vi "stiffnessSummaryView.vi"(10 "UserEvents in":refnum<class "UserEvents.lvclass">) -> ()   [LabVIEW 2015, in "M1M3SSSTViews.lvlib"]
uses:
  M1M3SSSTViews.lvlib
  UserEvents/UserEvents.lvclass
  UserEvents/UserEvents.lvclass/UserEvents.ctl
  Typedefs/StateSelector.ctl
  Typedefs/M1M3SSSTypedefs.lvlib
panel:
  in  "Stiffnesses Summary":string[][](table)
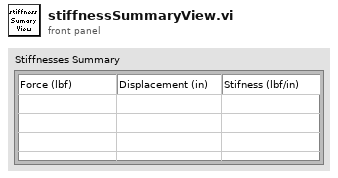
[diagram p1: front panel]
types:
  T1 = typedef "M1M3SSSTypedefs.lvlib/PubDataEvents.ctl" = cluster{"State":refnum<user-event>, "ErrorCode":refnum<user-event>, "OutputData":refnum<user-event>, "InputData":refnum<user-event>, "ControllerData":refnum<user-event>, "TestStatus":refnum<user-event>, "LogPath":refnum<user-event>, "StiffnessDataAssembly":refnum<user-event>, "PreconditioningCycle":refnum<user-event>}
  T2 = cluster{"Event Registration Refnum":refnum<event-registration>, "Event Registration Refnum":refnum<event-registration>}
  T3 = typedef "M1M3SSSTypedefs.lvlib/StateSelector.ctl" = enum16{"FaultState", "OffState", "RampingUpPressurePState", "RampingUpPressureSTState", "StandbyState", "StoppedState", "WaitingForSettledPState", "WaitingForSettledSTState"}
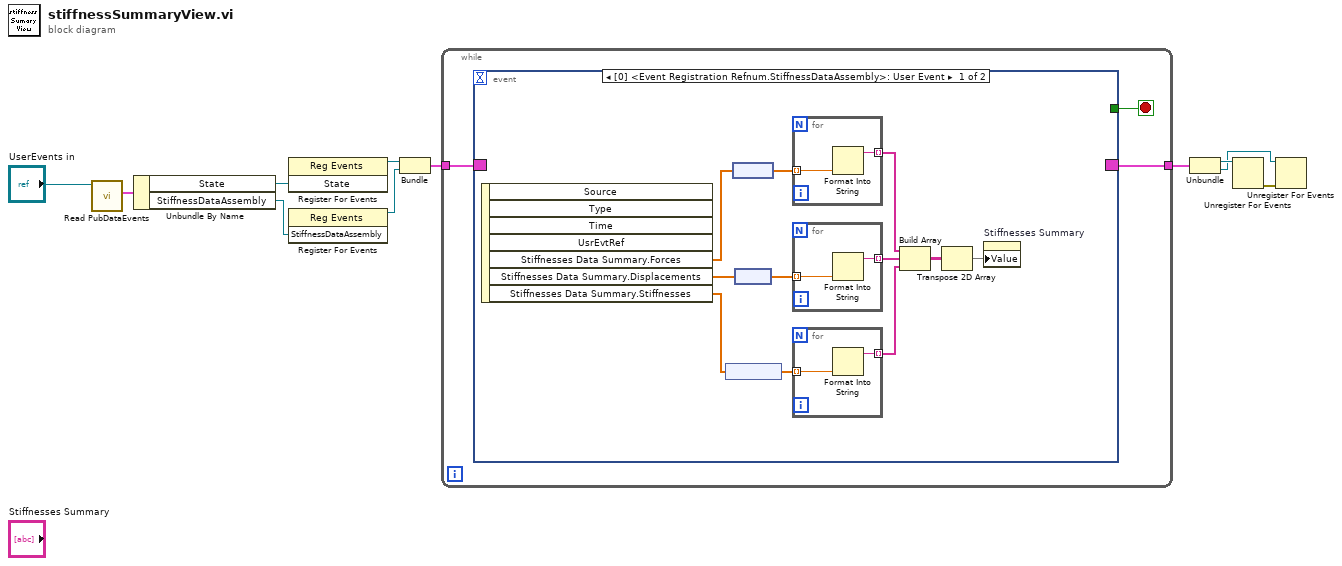
[diagram p0: block diagram]
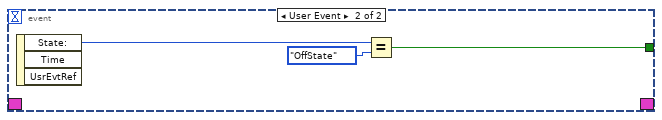
[diagram p2: hidden frame]
diagram:
  n1 = call "Read PubDataEvents.vi"("UserEvents in"="UserEvents in") -> ("PubDataEvents"=w11:T1)  [unwired: 9 in, 1 out]
  n2 = Unbundle By Name(w11) -> ("State"=w10:refnum<user-event>, "StiffnessDataAssembly"=w2:refnum<user-event>)
  n3 = register-events(w10) -> (reference out=w9:refnum<event-registration>)  [unwired: 2 in, 1 out]
  n4 = register-events(w2) -> (reference out=w1:refnum<event-registration>)  [unwired: 2 in, 1 out]
  n5 = Bundle("Event Registration Refnum"=w9, "Event Registration Refnum"=w1) -> (w7:T2)  [unwired: 1 in]
  n6 = while {
    tunnel: w7 -> [w14]
    tunnel: [w12] -> w6
    stop <- w13 stop-if-true
    n7 = event shown="[0] <Event Registration Refnum.StiffnessDataAssembly>: User Event" {
      selector: w14 -> [_ _]
      dyn-events: [_ _] -> w12
      timeout: _ -> [_ _]
      tunnel: [_ w33] -> w13
      event User Event {
        n8 = event-data() -> ("Stiffnesses Data Summary.Forces"=w22:dbl[unit][], "Stiffnesses Data Summary.Displacements"=w21:dbl[unit][], "Stiffnesses Data Summary.Stiffnesses"=w20:dbl[unit][])  [unwired: 1 in, 4 out]
        n9 = node(w20) -> (w23:dbl[])
        n10 = node(w22) -> (w24:dbl[])
        n11 = node(w21) -> (w25:dbl[])
        n12 = for {
          tunnel: w24 -> [w29] mode=indexing
          tunnel: [w28] -> w16 mode=indexing
          n13 = Format Into String(w29) -> (resulting string=w28:string)  [unwired: 3 in, 1 out]
        }
        n14 = for {
          tunnel: w25 -> [w31] mode=indexing
          tunnel: [w30] -> w15 mode=indexing
          n15 = Format Into String(w31) -> (resulting string=w30:string)  [unwired: 3 in, 1 out]
        }
        n16 = for {
          tunnel: w23 -> [w27] mode=indexing
          tunnel: [w26] -> w19 mode=indexing
          n17 = Format Into String(w27) -> (resulting string=w26:string)  [unwired: 3 in, 1 out]
        }
        n18 = Build Array(w16, w15, w19) -> (w18:string[][])
        n19 = Transpose 2D Array(2D array=w18) -> (transposed array=w17:string[][])
        n20 = property on="Stiffnesses Summary" class="Tbl (strict)"("Value"=w17) -> ()  [unwired: 2 in, 2 out]
      }
      event User Event {
        n21 = event-data() -> ("State:"=w32:T3)  [unwired: 1 in, 2 out]
        n22 = Equal?(x=w32, y=StateSelector."OffState" ("State:")) -> (x = y?=w33:bool)
      }
    }
  }
  n23 = Unbundle(w6) -> ("Event Registration Refnum"=w5:refnum<event-registration>, "Event Registration Refnum"=w4:refnum<event-registration>)
  n24 = Unregister For Events(event registration refnum=w5) -> (error out=w3:errorcluster)  [unwired: 1 in]
  n25 = Unregister For Events(event registration refnum=w4, error in=w3) -> ()  [unwired: 1 out]
